vi "Configure Instrument.vi"(8 "error in (no error)":errorcluster, 11 "Sequence Experiment":refnum<class "Control Experiment.lvclass">) -> (0 "error out":errorcluster, 3 "Sequence Experiment out":refnum<class "Control Experiment.lvclass">)   [LabVIEW 2016, in "Control Experiment.lvclass"]
uses:
  Control Experiment.lvclass
  <userlib>/LevyLab/Levylab Instruments/SMOs/Instrument/Instrument.lvclass
panel:
  # "Use this if you want to \nhave a configuration\nwindow specific to your\ninstrument. Otherwise you\nmay delete"
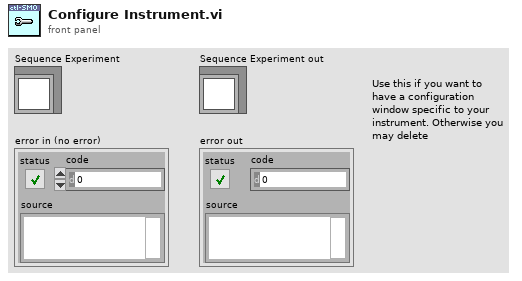
[diagram p1: front panel]
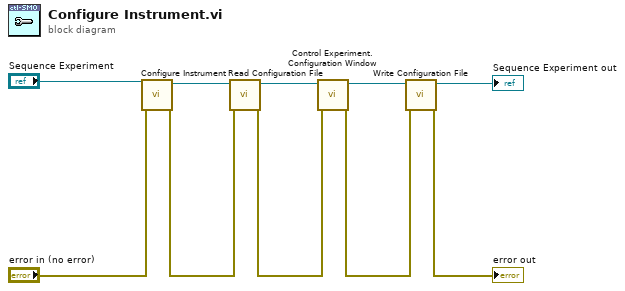
[diagram p0: block diagram]
diagram:
  n1 = call-parent "Configure Instrument.vi"("error in (no error)"="error in (no error)", "Instrument in"="Sequence Experiment") -> ("error out"=w5:errorcluster, "Instrument out"=w7:refnum<class "Control Experiment.lvclass">)  [unwired: 8 in]
  n2 = call-dynamic "Read Configuration File.vi"("error in (no error)"=w5, "Sequence Experiment"=w7) -> ("error out"=w4:errorcluster, "Sequence Experiment out"=w3:refnum<class "Control Experiment.lvclass">)  [unwired: 8 in]
  n3 = call "Control Experiment.Configuration Window.vi"("error in (no error)"=w4, "Sequence Experiment"=w3) -> ("error out"=w1:errorcluster, "Sequence Experiment out"=w2:refnum<class "Control Experiment.lvclass">)  [unwired: 8 in]
  n4 = call-dynamic "Write Configuration File.vi"("error in (no error)"=w1, "Sequence Experiment"=w2) -> ("error out"=→"error out":errorcluster, "Sequence Experiment out"=→"Sequence Experiment out":refnum<class "Control Experiment.lvclass">)  [unwired: 8 in]
